vi "Main.vi"() -> ()   [LabVIEW 2016]
uses:
  <vilib>/Math Plots/3D Math Plots/3D Surface/3D Surface XCtrl/3D Surface.xctl
panel:
  in  "Divs":i32=30
  out "Superficie":refnum<class "3D Plot Datatype.lvclass">[](xcontrol)
  out "Specs":dbl[][](graph)
  out "Molinetes":cluster{timestamp[], dbl[]}[](graph)
  out "Extensômetros":cluster{timestamp[], dbl[]}[](graph)
  in  "TestDir":path=path "L:/Documentos/Programas em LabVIEW/Programas funcionais/GradesSaltoCaxias/Data/01_ENSAIO" caption="Pasta do ensaio"
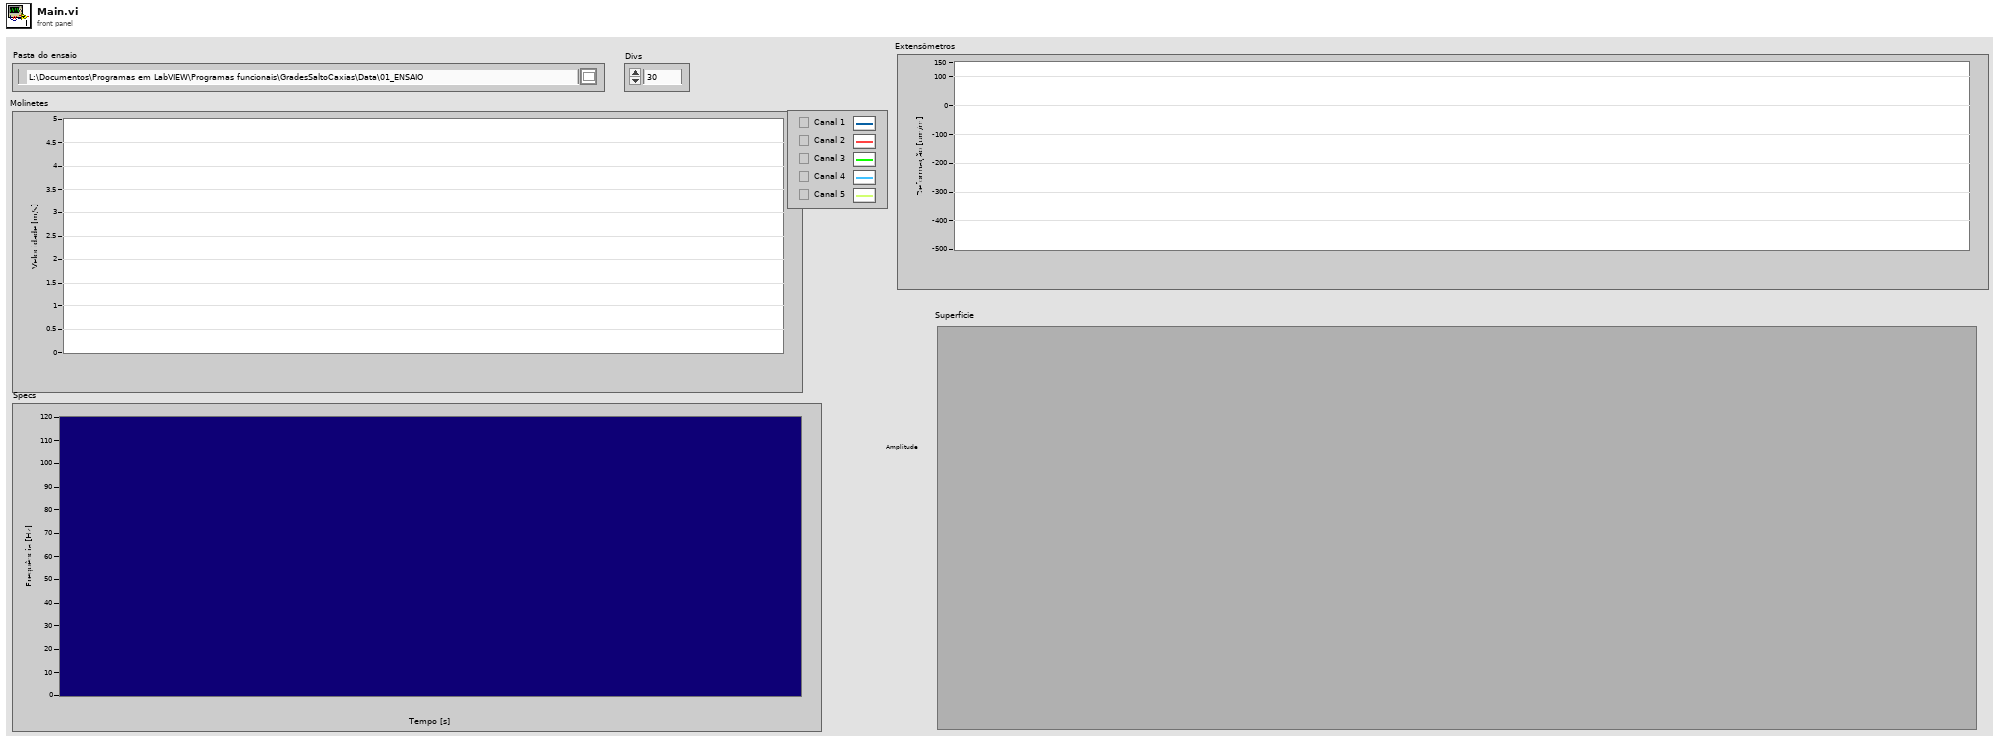
[diagram p1: front panel]
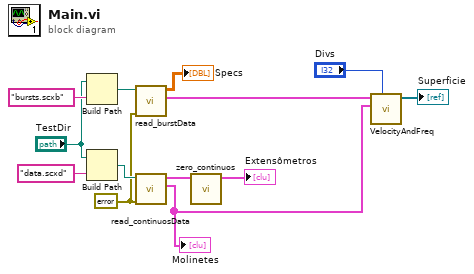
[diagram p0: block diagram]
diagram:
  w6 = errorcluster {"status"=FALSE, "code"=0, "source"=""} ("error in")
  n1 = Build Path(base path="TestDir", name or relative path="bursts.scxb") -> (appended path=w7:path)
  n2 = Build Path(base path="TestDir", name or relative path="data.scxd") -> (appended path=w12:path)
  n3 = call "read_burstData.vi"("error in"=w6, "DirPath"=w7) -> ("Specs_time"=w4:cluster{"Waveform":waveform(dbl), timestamp}[], "Specs"=→"Specs":dbl[][])  [unwired: 7 in, 1 out]
  n4 = call "read_continuosData.vi"("error in"=w6, "DirPath"=w12) -> ("CurrenMeters"=w3:cluster{"Array":timestamp[], "Array":dbl[]}[], "StrainGauges"=w11:cluster{"Array":timestamp[], "Array":dbl[]}[])  [unwired: 7 in, 1 out]
  "Molinetes" <- w3
  n5 = call "zero_continuos.vi"("StrainGauges"=w11) -> ("StrainGauges out"=→"Extensômetros":cluster{"Array":timestamp[], "Array":dbl[]}[])  [unwired: 10 in]
  n6 = call "VelocityAndFreq.vi"("Divs"="Divs", "CurrenMeters"=w3, "Specs_time"=w4) -> ("3D Plot lvclass Array out"=→"Superficie":refnum<class "3D Plot Datatype.lvclass">[])  [unwired: 8 in]
